vi "Set Custom Device Name.vi"(8 "error in (no error)":errorcluster, 10 "Custom Device Name":string, 11 "Project Sync Tools in":refnum<class "Project Sync Tools.lvclass">) -> (0 "error out":errorcluster, 3 "Project Sync Tools out":refnum<class "Project Sync Tools.lvclass">)   [LabVIEW 2019, in "Project Sync Tools.lvclass"]
uses:
  Project Sync Tools.lvclass
  Project Sync Tools.lvclass/Project Sync Tools.ctl
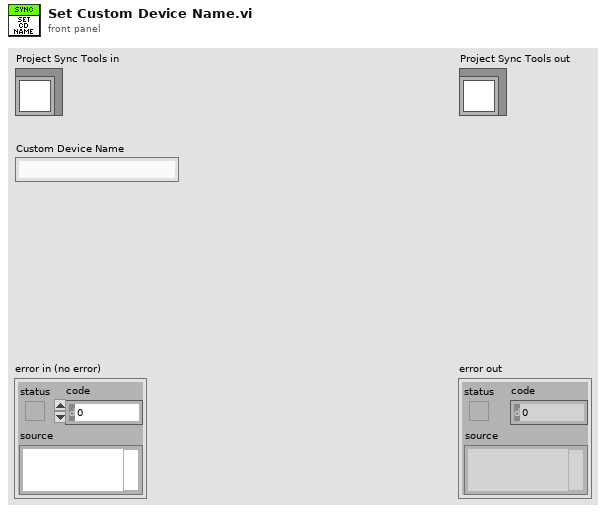
[diagram p1: front panel]
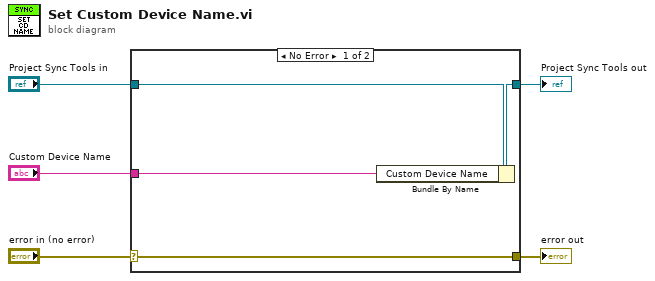
[diagram p0: block diagram]
diagram:
  n1 = case shown="No Error" "error in (no error)" {
    selector: "error in (no error)" -> [w9 w10]
    tunnel: [w9 w10] -> w4
    tunnel: [w7 w11] -> w2
    tunnel: "Project Sync Tools in" -> [w8 w11]
    tunnel: "Custom Device Name" -> [w6 _]
    frame No Error {
      n2 = Bundle By Name(cluster=w8, "Custom Device Name"=w6) -> (w7:refnum<class "Project Sync Tools.lvclass">)
    }
    frame Error {
    }
  }
  "error out" <- w4
  "Project Sync Tools out" <- w2
